vi "String2Bool.vi"(1 "字符串":string) -> (0 "布尔":bool)   [LabVIEW 2019]
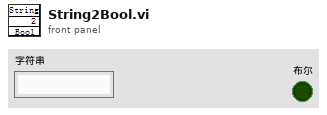
[diagram p1: front panel]
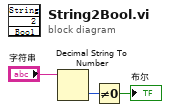
[diagram p0: block diagram]
diagram:
  n1 = Decimal String To Number(string="字符串") -> (number=w2:i32)  [unwired: 2 in, 1 out]
  n2 = Not Equal To 0?(x=w2) -> (x != 0?=→"布尔":bool)
